vi "Logfile.vi"() -> ()   [LabVIEW 2011]
uses:
  _GlobalVariables&Libraries/ATV Program Global Variables.vi
  <vilib>/Utility/file.llb/Write To Spreadsheet File (DBL).vi
panel:
  out "Navigation Duration(s)":i32
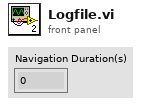
[diagram p1: front panel]
types:
  T1 = cluster{"End ATV Program":bool, "E-Stop":bool, "Save Logfile":bool, "Logfile Iteration Delay (ms)":u32, "Loop iteration time (ms)":u32, "Logfile Location":path, "Default GPS Navigation Path":path, "Computer":string, "Default GPS Boundary Path":path}
  T2 = cluster{"Obstacle Detected":bool, "Drive Speed":string, "Steer Angle":string, "Left Object":bool, "Right Object":bool, "Center Object":bool, "Rear Left":bool, "Rear Right":bool}
  T3 = cluster{"GPS VISA resource name":refnum<visa-resource-name>, "GPS Error":errorcluster, "Disable GPS VISA":bool, "Latitude":dbl, "Longitude":dbl, "Latitude Uncertainty":dbl, "Longitude Uncertainty":dbl, "GPS Signal":u32}
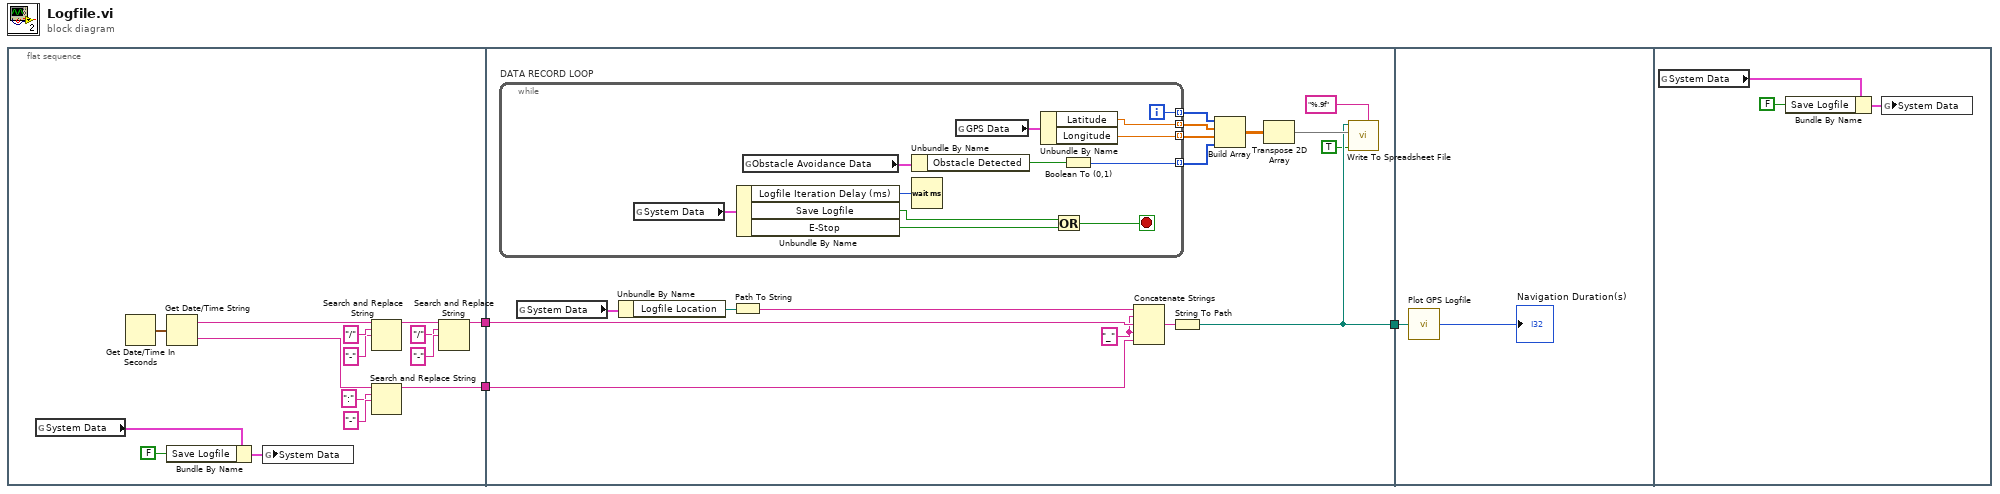
[diagram p0: block diagram]
diagram:
  n1 = flat-sequence {
    tunnel: [w8] -> w3
    tunnel: [w5] -> w1
    tunnel: w3 -> [w23]
    tunnel: [w22] -> w2
    tunnel: w1 -> [w28]
    tunnel: w2 -> [w48]
    frame #0 {
      n2 = global read "ATV Program Global Variables.vi" "System Data"() -> (w18:T1)
      n3 = Get Date/Time In Seconds() -> (seconds since 1Jan1904=w15:timestamp)
      n4 = Get Date/Time String(seconds (now)=w15) -> (date string=w12:string, time string=w9:string)  [unwired: 2 in]
      n5 = Bundle By Name(cluster=w18, "Save Logfile"=FALSE) -> (w17:T1)
      n6 = global write "ATV Program Global Variables.vi" "System Data"(w17) -> ()
      n7 = Search and Replace String(input string=w12, search string="/", replace string="-" ("replace string (\"\")")) -> (result string=w6:string)  [unwired: 5 in, 3 out]
      n8 = Search and Replace String(input string=w9, search string=":", replace string="-" ("replace string (\"\")")) -> (result string=w8:string)  [unwired: 5 in, 3 out]
      n9 = Search and Replace String(input string=w6, search string="/", replace string="-" ("replace string (\"\")")) -> (result string=w5:string)  [unwired: 5 in, 3 out]
    }
    frame #1 {
      w24 = "_" ("string")
      n10 = while "DATA RECORD LOOP" {
        tunnel: [w43] -> w34 mode=indexing
        tunnel: [w42] -> w33 mode=indexing
        tunnel: [w38] -> w29 mode=indexing
        tunnel: [w37] -> w20 mode=indexing
        i -> [w38]
        stop <- w41 stop-if-true
        n11 = global read "ATV Program Global Variables.vi" "System Data"() -> (w46:T1)
        n12 = Unbundle By Name(w46) -> ("Logfile Iteration Delay (ms)"=w45:u32, "Save Logfile"=w40:bool, "E-Stop"=w39:bool)
        n13 = global read "ATV Program Global Variables.vi" "Obstacle Avoidance Data"() -> (w36:T2)
        n14 = Unbundle By Name(w36) -> ("Obstacle Detected"=w35:bool)
        n15 = Wait (ms)(milliseconds to wait=w45) -> ()  [unwired: 1 out]
        n16 = global read "ATV Program Global Variables.vi" "GPS Data"() -> (w44:T3)
        n17 = Unbundle By Name(w44) -> ("Latitude"=w43:dbl, "Longitude"=w42:dbl)
        n18 = Or(x=w40, y=w39) -> (x .or. y?=w41:bool)
        n19 = Boolean To (0,1)(Boolean=w35) -> (0, 1=w37:i16)
      }
      n20 = global read "ATV Program Global Variables.vi" "System Data"() -> (w30:T1)
      n21 = Unbundle By Name(w30) -> ("Logfile Location"=w27:path)
      n22 = Path To String(path=w27) -> (string=w26:string)
      n23 = Concatenate Strings(w26, w24, w28, w24, w23) -> (w25:string)
      n24 = String To Path(string=w25) -> (path=w22:path)
      n25 = Build Array(w29, w34, w33, w20) -> (w19:dbl[][])
      n26 = Transpose 2D Array(2D array=w19) -> (transposed array=w32:dbl[][])
      n27 = call-poly <vilib>:"Write To Spreadsheet File.vi"("format (%.3f)"="%.9f", "append to file? (new file:F)"=TRUE, "2D data"=w32, "file path (dialog if empty)"=w22) -> ()  [unwired: 4 in, 1 out]
    }
    frame #2 {
      n28 = call "Plot GPS Logfile.vi"("file path (dialog if empty)"=w48) -> ("Navigation Duration(s)"=→"Navigation Duration(s)":i32)
    }
    frame #3 {
      n29 = global read "ATV Program Global Variables.vi" "System Data"() -> (w49:T1)
      n30 = Bundle By Name(cluster=w49, "Save Logfile"=FALSE) -> (w50:T1)
      n31 = global write "ATV Program Global Variables.vi" "System Data"(w50) -> ()
    }
  }
